vi "shortcut menu items.vi"(8 "selected":i32, 9 "channel names":string[](array[string]), 11 "Menu in":refnum<k9>) -> ()   [LabVIEW 2018]
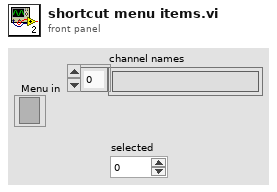
[diagram p1: front panel]
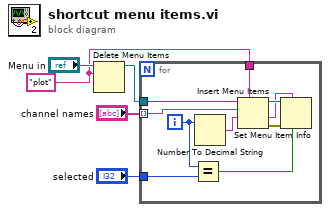
[diagram p0: block diagram]
diagram:
  w1 = "plot" ("menu tag")
  n1 = Delete Menu Items(8:w1, 9:"Menu in") -> (3:w2:refnum<k9>)  [unwired: 2 in, 1 out]
  n2 = for {
    tunnel: "channel names" -> [w12] mode=indexing
    tunnel: "selected" -> [w14]
    tunnel: w2 -> [w13]
    tunnel: w1 -> [w6]
    i -> [w15]
    n3 = Equal?(x=w15, y=w14) -> (x = y?=w7:bool)
    n4 = Number To Decimal String(number=w15) -> (decimal integer string=w11:string)  [unwired: 1 in]
    n5 = Insert Menu Items(5:w6, 7:w11, 8:w12, 9:w13) -> (0:w10:errorcluster, 1:w8:string, 3:w9:refnum<k9>)  [unwired: 2 in]
    n6 = Set Menu Item Info(6:w7, 7:w8, 8:w10, 11:w9) -> ()  [unwired: 3 in, 2 out]
  }
